vi "sv_Get Even-Angle Signal.vi"(0 "data to process":waveform(dbl)[](array[waveform]), 2 "reset?":bool, 11 "error in (no error)":errorcluster, 12 "maximum harmonic":i32=-1) -> (4 "data to process out":waveform(dbl)[](array[waveform]), 6 "even-angle signals":cluster{"r0":dbl, "dr":dbl, "Y":dbl[]}[](array[cluster]), 8 "even-angle channel info":T1[](array[typedef]) {"channel info"."pregain" format="%.2f"; "channel info"."weighting filter" items=["Linear", "A-weighting", "B-weighting", "C-weighting", "ITU-R 468-4", "Dolby", "CCITT", "C-message", "Wb", "Wc", "Wd", "We", "Wf", "Wh", "Wj", "Wk", "Wm", "AES17 20 kHz lowpass", "AES17 40 kHz lowpass", "AES17 20 kHz highpass", "AES17 40 kHz highpass"]; "channel info"."dB reference" format="%^.1e"; "channel info"."engineering units" items=["custom..."=0, "V"=1, "A"=21, "C"=30, "pC"=31, "s"=32, "-"=29, "Pa"=2, "N"=20, "g"=3, "m/s^2"=4, "m/s"=5, "m"=6, "mm/s"=12, "mm"=13, "micron/s"=14, "micron"=15, "in/s^2"=7, "in/s"=8, "in"=9, "mil/s"=10, "mil"=11, "rad/s^2"=16, "rad/s"=17, "rad"=18, "deg/s^2"=26, "deg/s"=27, "deg"=28, "RPM"=22, "cycle/s^2"=23, "Hz"=24, "cycle"=25, "strain"=19]; "channel info"."sensor sensitivity" format="%#_5f"}, 10 "even-angle position info":T5, 14 "actual maximum harmonic":i32=-1, 15 "error out":errorcluster)   [LabVIEW 2017, in "SoundVib_ContSweptSine.lvlib"]
uses:
  <vilib>/addons/Sound and Vibration/svt_Continuous Swept Sine/SoundVib_ContSweptSine.lvlib
  <vilib>/addons/Sound and Vibration/Order Analysis/Misc/OAT Position Info.ctl
  <vilib>/addons/_NISVFA/_Shared subVIs/Controls/svc_Resampled Channel Info.ctl
  <vilib>/addons/_NISVFA/_Shared subVIs/Controls/svc_Channel Info.ctl
  <vilib>/addons/_NISVFA/_Shared subVIs/Controls/svc_Engineering Units Text Ring.ctl
  <vilib>/addons/_NISVFA/_Shared subVIs/Controls/svc_Weighting Filter Text Ring.ctl
  <vilib>/addons/Sound and Vibration/svt_Continuous Swept Sine/subVIs/sv_Continuous Swept-Sine Tags.ctl
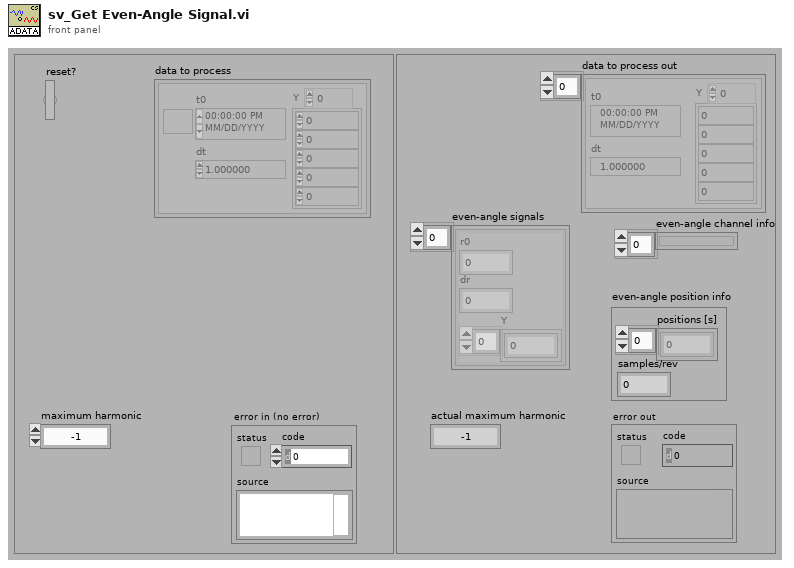
[diagram p1: front panel]
types:
  T1 = typedef "svc_Resampled Channel Info.ctl" = cluster{"channel name":string, "description":string, " channel info":T2}
  T2 = typedef "svc_Channel Info.ctl" = cluster{"sensor sensitivity":dbl, "engineering units":T3, "dB reference":dbl, "custom label":string, "weighting filter":T4, "pregain":dbl}
  T3 = typedef "svc_Engineering Units Text Ring.ctl" = u16
  T4 = typedef "svc_Weighting Filter Text Ring.ctl" = u16
  T5 = typedef "OAT Position Info.ctl" = cluster{"positions [s]":dbl[], "samples/rev":dbl}
  T6 = typedef "SoundVib_ContSweptSine.lvlib/sv_Continuous Swept-Sine Tags.ctl" = enum16{"samplesPerRevolution", "t2aPositions", "a2tPositions", "evenAngleSignal", "evenAnglePositionInfo", "evenAngleChannelInfo"}
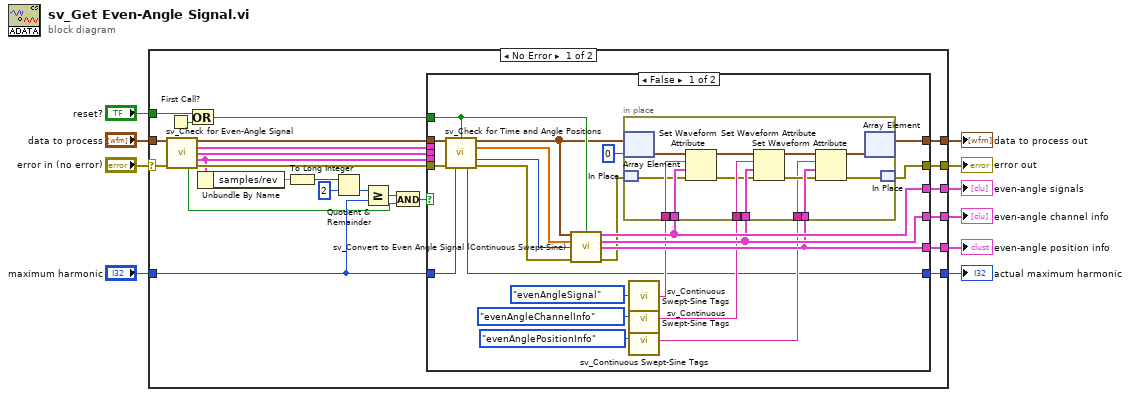
[diagram p0: block diagram]
diagram:
  n1 = case shown="No Error" "error in (no error)" {
    selector: "error in (no error)" -> [w33 w78]
    tunnel: [w27 w78] -> w9
    tunnel: "data to process" -> [w34 w77]
    tunnel: [w28 w77] -> w7
    tunnel: [w26 _] -> w6
    tunnel: [w25 _] -> w5
    tunnel: [w24 _] -> w4
    tunnel: "reset?" -> [w22 _]
    tunnel: "maximum harmonic" -> [w14 _]
    tunnel: [w13 _] -> w1
    frame No Error {
      n2 = First Call?() -> (First Call?: T/F=w23:bool)
      n3 = call <vilib>:"sv_Check for Even-Angle Signal.vi"("data to process"=w34, "error in (no error)"=w33) -> ("data to process out"=w32:waveform(dbl)[], "even-angle signals"=w31:cluster{"r0":dbl, "dr":dbl, "Y":dbl[]}[], "even-angle channel info"=w30:T1[], "even-angle position info"=w20:T5, "found"=w11:bool, "error out"=w29:errorcluster)  [unwired: 8 in]
      n4 = Or(x=w22, y=w23) -> (x .or. y?=w21:bool)
      n5 = Unbundle By Name(w20) -> ("samples/rev"=w18:dbl)
      n6 = To Long Integer(number=w18) -> (32bit integer=w17:i32)
      n7 = Quotient & Remainder(x=w17, y=2) -> (floor(x/y)=w12:i32)  [unwired: 1 out]
      n8 = Greater Or Equal?(x=w12, y=w14) -> (x >= y?=w15:bool)
      n9 = And(x=w15, y=w11) -> (x .and. y?=w19:bool)
      n10 = case shown="False" w19 {
        tunnel: w32 -> [w56 w76]
        tunnel: w31 -> [_ w75]
        tunnel: w30 -> [_ w74]
        tunnel: w20 -> [_ w73]
        tunnel: w29 -> [w55 w72]
        tunnel: w21 -> [w53 _]
        tunnel: [w38 w76] -> w28
        tunnel: [w50 w75] -> w26
        tunnel: [w49 w74] -> w25
        tunnel: [w48 w73] -> w24
        tunnel: [w39 w72] -> w27
        tunnel: w14 -> [w36 w71]
        tunnel: [w35 w71] -> w13
        frame False {
          n11 = call <vilib>:"sv_Check for Time and Angle Positions.vi"("data to process"=w56, "reset?"=w53, "error in (no error)"=w55, "harmonic"=w36) -> ("data to process out"=w41:waveform(dbl)[], "time array [s]"=w52:dbl[], "samples/rev"=w51:i32, "actual harmonic"=w35:i32, "error out"=w54:errorcluster)  [unwired: 6 in, 1 out]
          n12 = call <vilib>:"sv_Convert to Even Angle Signal (Continuous Swept-Sine).vi"("scaled signals [EU]"=w41, "reset? (F)"=w53, "new sample time [s]"=w52, "new samples/rev"=w51, "error in (no error)"=w54) -> ("even-angle signals"=w50:cluster{"r0":dbl, "dr":dbl, "Y":dbl[]}[], "even-angle channel info"=w49:T1[], "even-angle position info"=w48:T5, "error out"=w40:errorcluster)  [unwired: 6 in, 1 out]
          n13 = call <vilib>:"sv_Continuous Swept-Sine Tags.vi"("chirp sweep tag selector"=sv_Continuous_Swept-Sine_Tags."evenAngleSignal") -> ("Tag"=w46:string)
          n14 = call <vilib>:"sv_Continuous Swept-Sine Tags.vi"("chirp sweep tag selector"=sv_Continuous_Swept-Sine_Tags."evenAngleChannelInfo") -> ("Tag"=w44:string)
          n15 = call <vilib>:"sv_Continuous Swept-Sine Tags.vi"("chirp sweep tag selector"=sv_Continuous_Swept-Sine_Tags."evenAnglePositionInfo") -> ("Tag"=w42:string)
          n16 = in-place {
            in-place-border: w50 -> [w70]
            in-place-border: w49 -> [w69]
            in-place-border: w48 -> [w68]
            in-place-border: w46 -> [w67]
            in-place-border: w44 -> [w63]
            in-place-border: w42 -> [w62]
            n17 = in-place-array #1(w41, 0) -> (w60:waveform(dbl))
            n18 = in-place-match #2(w40) -> (w58:errorcluster)
            n19 = Set Waveform Attribute(4:w58, 5:w70, 6:w67, 7:w60) -> (0:w61:errorcluster, 3:w66:waveform(dbl))  [unwired: 1 out]
            n20 = Set Waveform Attribute(4:w61, 5:w69, 6:w63, 7:w66) -> (0:w65:errorcluster, 3:w64:waveform(dbl))  [unwired: 1 out]
            n21 = Set Waveform Attribute(4:w65, 5:w68, 6:w62, 7:w64) -> (0:w57:errorcluster, 3:w59:waveform(dbl))  [unwired: 1 out]
            n22 = in-place-array #1(w59) -> (w38:waveform(dbl)[])  [unwired: 1 out]
            n23 = in-place-match #2(w57) -> (w39:errorcluster)
          }
        }
        frame True {
        }
      }
    }
    frame Error {
    }
  }
  "error out" <- w9
  "even-angle signals" <- w6
  "even-angle position info" <- w4
  "even-angle channel info" <- w5
  "data to process out" <- w7
  "actual maximum harmonic" <- w1
